vi "qWGC.vi"(0 "System no.":i32=1 min=1 max=4 step=1, 2 "Axes to query":string[](array[string]), 3 "All axes?":bool, 4 "Axis identifier?":bool=TRUE, 5 "error in":errorcluster) -> (14 "Cycles":i32[](array[numeric]), 19 "error out":errorcluster)   [LabVIEW 2026]
doc: "Returns number of wave generator cycles set for specified axes.\n\nC-413: Axes to query is identical with wave generator ID, which can be 1 to 2. All axes? = must be FALSE. \n\nC-886: Axes to query is identical with wave generator ID, which can be 1 to No. of connected axes. All axes? = must be FALSE.\n\nC-887: Axes to query is identical with wave generator ID, which can be 1 to No. of connected axes. All axes? = must be FALSE.\n\nC-891: Axes to query is identical with wave generator ID, which can be 1. All axes? = must be FALSE. \n\nE-516: If All axes = TRUE, then Axis identifier must be TRUE\n\nE-517, E-518: Axes to query is identical with wave generator ID, which can be 1 to 3. All axes? must be FALSE.\n\nE-709: Axes to query is identical with wave generator ID, which can be 1. All axes? must be FALSE.\n\nE-712: Axes to query is identical with wave generator ID, which can be 1 to No. of connected axes. All axes? must be FALSE.\n\nE-725, E-727: Axes to query is identical with wave generator ID, which can be 1 to No. of connected axes. All axes? must be FALSE.\n\nE-753: Axes to query is identical with wave generator ID, which can be 1. All axes? must be FALSE.\n\nE-754: Axes to query is identical with wave generator ID, which can be 1. All axes? must be FALSE.\n\nE-761: Axes to query is identical with wave table number, which can be 1 to 4. All axes must be FALSE"
panel:
  # "Returns number of wave generator cycles set for specified axes."
  # "If all axes: use"
  # "Query"
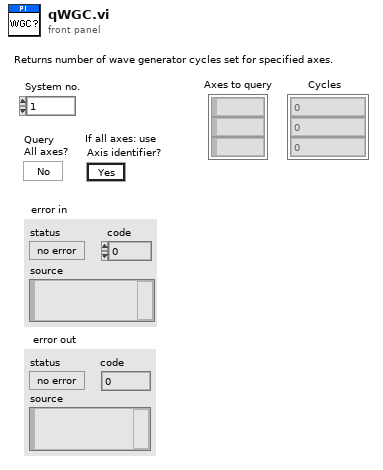
[diagram p1: front panel]
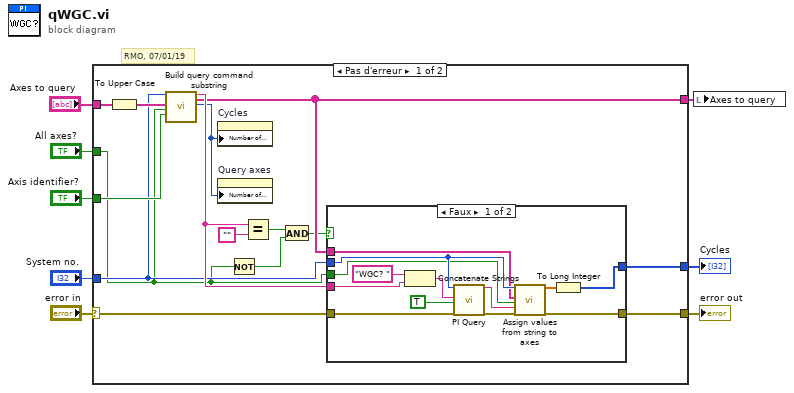
[diagram p0: block diagram]
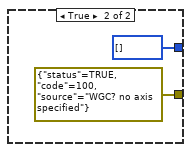
[diagram p2: hidden frame]
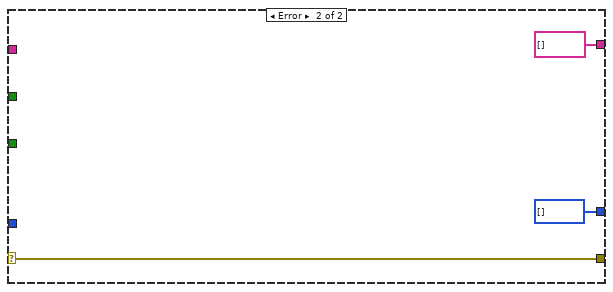
[diagram p3: hidden frame]
diagram:
  # "RMO, 07/01/19"
  n1 = case shown="Pas d'erreur" "error in" {
    selector: "error in" -> [w9 w40]
    tunnel: [w23 i32[] []] -> w8
    tunnel: "Axes to query" -> [w22 _]
    tunnel: [w11 w40] -> w6
    tunnel: "Axis identifier?" -> [w19 _]
    tunnel: "System no." -> [w16 _]
    tunnel: [w15 string[] [] ("Axes to query out")] -> w3
    tunnel: "All axes?" -> [w14 _]
    frame No Error {
      n2 = To Upper Case(1:w22) -> (0:w20:string[])
      n3 = call "Build query command substring.vi"("System no."=w16, "Axes to query in"=w20, "Query\nAll axes?"=w14, "For all axes: use\nAxis identifier?"=w19) -> ("Command substring"=w18:string, "Axes to query out"=w15:string[], "Number of rows"=w17:u32)  [unwired: 2 in, 11 out]
      n4 = property on="Cycles" class="Tabl (strict)"("Number of Rows"=w17) -> ()  [unwired: 2 in, 2 out]
      n5 = property on="Query axes" class="Tabl (strict)"("Number of Rows"=w17) -> ()  [unwired: 2 in, 2 out]
      n6 = Not(x=w14) -> (.not. x?=w12:bool)
      n7 = Equal?(x=w18, y="" ("x")) -> (x = y?=w13:bool)
      n8 = And(x=w13, y=w12) -> (x .and. y?=w10:bool)
      n9 = case shown="Faux" w10 {
        tunnel: [w26 i32[] []] -> w23
        tunnel: w18 -> [w33 _]
        tunnel: w16 -> [w32 _]
        tunnel: w15 -> [w31 _]
        tunnel: w14 -> [w30 _]
        tunnel: w9 -> [w29 _]
        tunnel: [w28 errorcluster {"status"=TRUE, "code"=100, "source"="WGC? no axis specified"} ("error out")] -> w11
        frame False {
          n10 = Concatenate Strings("WGC? ", w33) -> (w34:string)
          n11 = call "PI Query.vi"("System no."=w32, "String to send"=w34, "Attach termination char.?"=TRUE ("Attach Linefeed?"), "error in"=w29) -> ("String read"=w25:string, "error out"=w24:errorcluster)  [unwired: 3 in, 11 out]
          n12 = call "Assign values from string to axes.vi"("System no."=w32, "Queried axes"=w31, "All axes queried?"=w30, "Input String"=w25, "error in"=w24) -> ("Values"=w27:dbl[], "error out"=w28:errorcluster)  [unwired: 4 in, 9 out]
          n13 = To Long Integer(number=w27) -> (32bit integer=w26:i32[])
        }
        frame True {
        }
      }
    }
    frame Error {
    }
  }
  "error out" <- w6
  "Cycles" <- w8
  n14 = local write "Axes to query"(w3) -> ()
